vi "VNA Client.vi"(8 "error in (no error)":errorcluster, 9 "Data":variant, 10 "Command":string, 11 "VNA in":refnum<class "VNA.lvclass">) -> (0 "error out":errorcluster, 3 "VNA out":refnum<class "VNA.lvclass">)   [LabVIEW 2016, in "VNA.lvclass"]
uses:
  VNA.lvclass
  C:/Program Files (x86)/National Instruments/LabVIEW 2016/user.lib/LevyLab/Levylab Instruments/SMOs/Instrument/Instrument.lvclass
  <userlib>/LevyLab/Levylab Instruments/SMOs/Instrument/Typedefs/SMO Configuration--Cluster.ctl
  <userlib>/LevyLab/Levylab Instruments/SMOs/Instrument/Typedefs/SMO RC Type--enum.ctl
  <userlib>/LevyLab/Levylab Instruments/SMOs/Instrument/Instrument.lvclass/Instrument.ctl
  <userlib>/LevyLab/Levylab Instruments/SMOs/Instrument/Instrument.lvclass
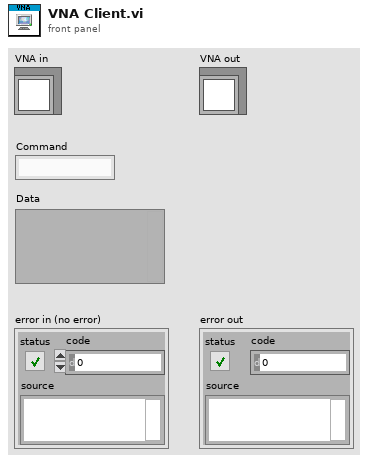
[diagram p1: front panel]
types:
  T1 = typedef "Instrument.lvclass/SMO Configuration--Cluster.ctl" = cluster{"Address":string, "Port":u16, "RC Type":T2}
  T2 = typedef "Instrument.lvclass/SMO RC Type--enum.ctl" = enum16{"RC", "STM", "ZMQ"}
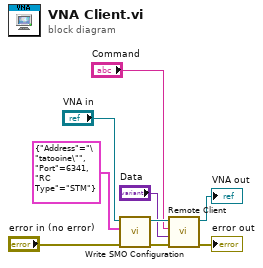
[diagram p0: block diagram]
diagram:
  n1 = call <userlib>:"Write SMO Configuration.vi"("error in (no error)"="error in (no error)", "SMO"=T1 {"Address"="\"tatooine\"", "Port"=6341, "RC Type"=enum."STM"}, "Instrument in"="VNA in") -> ("error out"=w8:errorcluster, "Instrument out"=w6:refnum<class "VNA.lvclass">)  [unwired: 7 in]
  n2 = call-dynamic "Remote Client.vi"("error in (no error)"=w8, "Data"="Data", "Command"="Command", "Instrument in"=w6) -> ("error out"=→"error out":errorcluster, "Instrument out"=→"VNA out":refnum<class "VNA.lvclass">)  [unwired: 4 in, 2 out]
